vi "ExecuteMenuCommand.vi"(0 "reference in":refnum<class "InterfaceNode.lvclass">, 1 "Command":string, 5 "error in (no error)":errorcluster) -> (14 "reference out":refnum<class "InterfaceNode.lvclass">, 15 "EditorAction":T3, 16 "FlattenCommandSettings":T1, 19 "error out":errorcluster)   [LabVIEW 2020, in "InterfaceNode.lvclass"]
uses:
  <resource>/Framework/Providers/Open_GDS/UML/InterfaceNode_class/InterfaceNode.lvclass
  <resource>/Framework/Providers/Open_GDS/UML/UMLEditor/UMLEditor EditorActionType.ctl
  <resource>/Framework/Providers/Open_GDS/UML/UMLEditor/UMLEditor FlattenCommandType.ctl
  <resource>/Framework/Providers/Open_GDS/UML/UMLEditor/UMLEditor ExecuteCommandType.ctl
  <resource>/Framework/Providers/Open_GDS/UML/ClassNode_class/ClassNode.lvclass
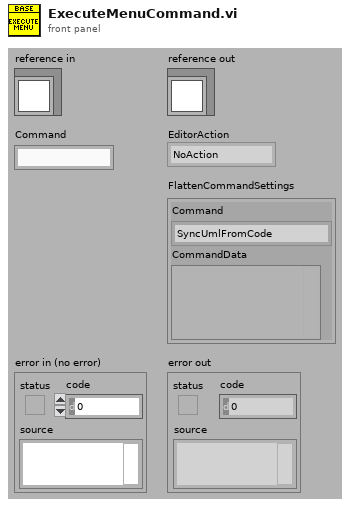
[diagram p1: front panel]
types:
  T1 = typedef "UMLEditor FlattenCommandType.ctl" = cluster{"Command":T2, "CommandData":variant}
  T2 = typedef "UMLEditor ExecuteCommandType.ctl" = enum16{"SyncUmlFromCode", "SyncCodeFromUML", "OpenClass", "OpenFile", "CreateClass", "CreateVI", "OpenClassAttribute", "LocateInProject", "GraphExecute"}
  T3 = typedef "UMLEditor EditorActionType.ctl" = enum16{"NoAction", "Repaint", "ExecuteCommand"}
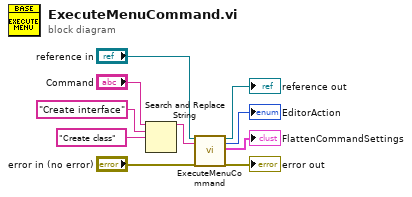
[diagram p0: block diagram]
diagram:
  n1 = Search and Replace String(input string="Command", search string="Create interface", replace string="Create class" ("search string")) -> (result string=w1:string)  [unwired: 5 in, 3 out]
  n2 = call-parent "ExecuteMenuCommand.vi"("reference"="reference in", "Command"=w1, "error in (no error)"="error in (no error)") -> ("reference out"=→"reference out":refnum<class "InterfaceNode.lvclass">, "EditorAction"=→"EditorAction":T3, "FlattenCommandSettings"=→"FlattenCommandSettings":T1, "error out"=→"error out":errorcluster)  [unwired: 13 in]
